vi "from string.vi"(8 "error in":errorcluster, 9 "data":string, 10 "version":string, 11 "fixed channel configuration in":refnum<class "DAQmx Watchdog configuration.lvclass">) -> (0 "error out":errorcluster, 3 "fixed channel configuration out":refnum<class "DAQmx Watchdog configuration.lvclass">)   [LabVIEW 2014, in "DAQmx Watchdog configuration.lvclass"]
doc: "Provides an interface for loading a module configuration from a file or other serialized data source. It is recommended that all children of this class store data in two sets--data required for its own initialization, and any data required for parent initialization--and that each implementation uses the <b>Call Parent Method</b> primitive to de-serialize parent information. As a result, it is expected that every module configuration class calls <b>component configuration.lvclass:From String.vi</b>.\nNI Tag Bus Module Framework 1.0.3.43\nNI Systems Engineering"
uses:
  DAQmx Watchdog configuration.lvclass
  <vilib>/NI/DCAF/Tag Editor Core/control module/configuration/control module configuration.lvclass
  <vilib>/NI/Configuration Framework/serializable configuration/NISE_CEF_serializable configuration.lvclass
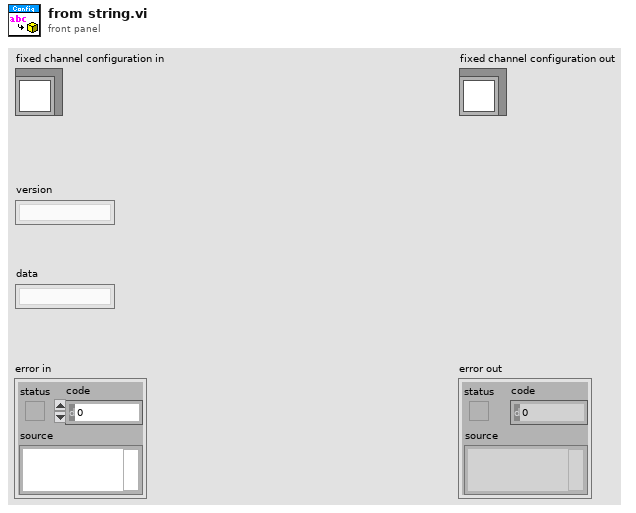
[diagram p1: front panel]
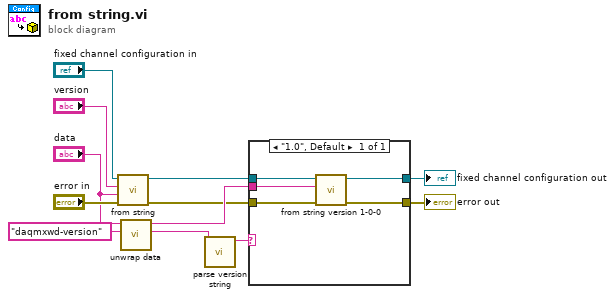
[diagram p0: block diagram]
diagram:
  n1 = call-parent "from string.vi"("error in"="error in", "data"="data", "version"="version", "fixed channel configuration in"="fixed channel configuration in") -> ("error out"=w2:errorcluster, "fixed channel configuration out"=w4:refnum<class "DAQmx Watchdog configuration.lvclass">)  [unwired: 6 in]
  n2 = call <vilib>:"unwrap data.vi"("identifier"="daqmxwd-version", "data to unwrap"="data") -> ("unwrapped data"=w7:string, "remaining string"=w5:string)  [unwired: 8 in]
  n3 = call <vilib>:"parse version string.vi"("full version"=w7) -> ("major.minor version"=w6:string)  [unwired: 7 in, 3 out]
  n4 = case shown="\"1.0\", Default" w6 {
    tunnel: w5 -> [w17]
    tunnel: w4 -> [w16]
    tunnel: [w15] -> w3
    tunnel: w2 -> [w14]
    tunnel: [w13] -> w1
    frame "1.0", Default {
      n5 = call "from string version 1-0-0.vi"("error in (no error)"=w14, "Data String"=w17, "DAQmx Watchdog configuration in"=w16) -> ("error out"=w13:errorcluster, "DAQmx Watchdog configuration out"=w15:refnum<class "DAQmx Watchdog configuration.lvclass">)  [unwired: 7 in]
    }
  }
  "error out" <- w1
  "fixed channel configuration out" <- w3
